vi "DAQmx Task State Model Benchmark.vi"() -> ()   [LabVIEW 2010]
doc: "Description:\nThis VI explores the differences in timing within a VI depending on how the DAQmx Task State is set before running a DAQmx Read VI.\n\nInstructions:\n1. Set the physical channels control to any analog input channel\n2. Run the VI\n3. Observe the different amounts of time the DAQmx Read takes depending upon which State the DAQmx Task was in before the read operation."
uses:
  DAQmx Task States.ctl
  <vilib>/DAQmx/read.llb/DAQmx Read (Analog 1D DBL 1Chan NSamp).vi
  <vilib>/DAQmx/create/channels.llb/DAQmx Create Channel (AI-Voltage-Basic).vi
  <vilib>/daqmx/miscellaneous.llb/DAQmx Fill In Error Info.vi
panel:
  out "Running Task Progress":i32(slide) scale=0.0..100.0
  out "Running Task (ms/iteration)":dbl max=10.0 format="%.2f"
  out "Committed Task Progress":i32(slide) scale=0.0..100.0
  out "Committed Task (ms/iteration)":dbl max=10.0 format="%.2f"
  out "Reserved Task Progress":i32(slide) scale=0.0..100.0
  out "Reserved Task (ms/iteration)":dbl max=10.0 format="%.2f"
  out "Verified Task Progress":i32(slide) scale=0.0..100.0
  out "Verified Task (ms/iteration)":dbl max=10.0 format="%.2f"
  in  "Iterations":i32=100
  out "Unverified Task Progress":i32(slide) scale=0.0..100.0
  out "Unverified Task (ms/iteration)":dbl max=10.0 format="%.2f"
  in  "physical channels":tag
  # "Directions:\n1.  Set the physical channels control to any analog input channel\n2.  Set the number of iterations to the desired number (10 < i < 1000)\n3.  Run the VI\n4.  Observe the difference in execution times depending upon which DAQmx Task State is set before the DAQmx Read.\n\nNote: Each DAQmx Read must continue throught the DAQmx Task States and get to Running before any data can be returned."
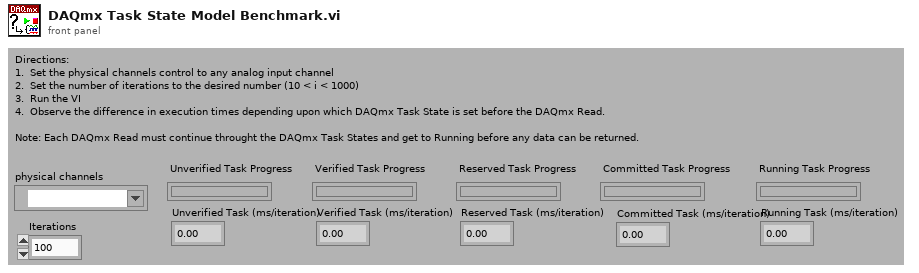
[diagram p1: front panel]
types:
  T1 = typedef "DAQmx Task States.ctl" = enum16{"Unverified", "Verified", "Reserved", "Committed", "Running"}
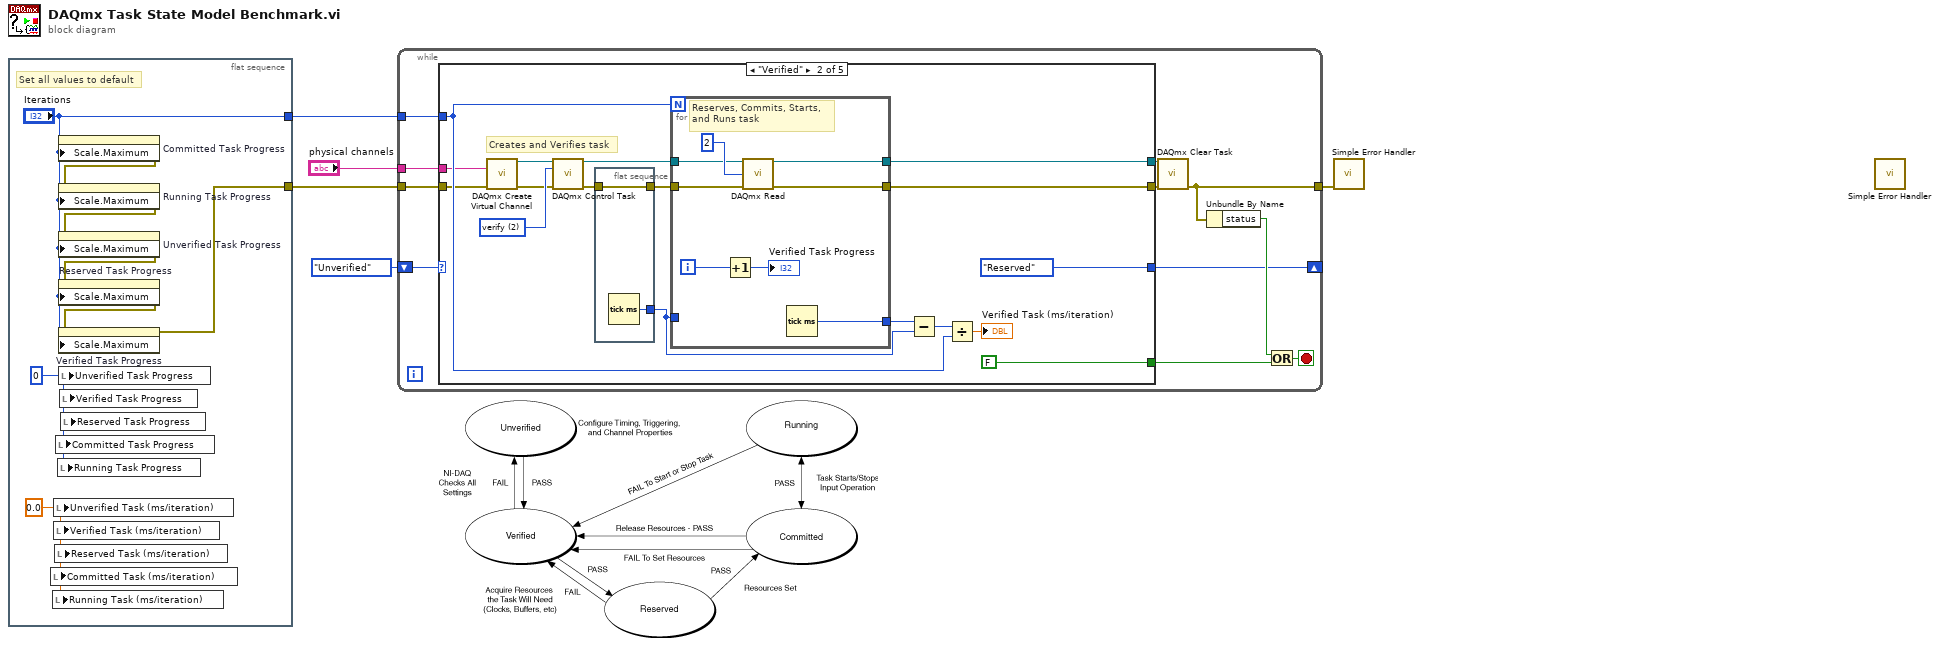
[diagram p0: block diagram]
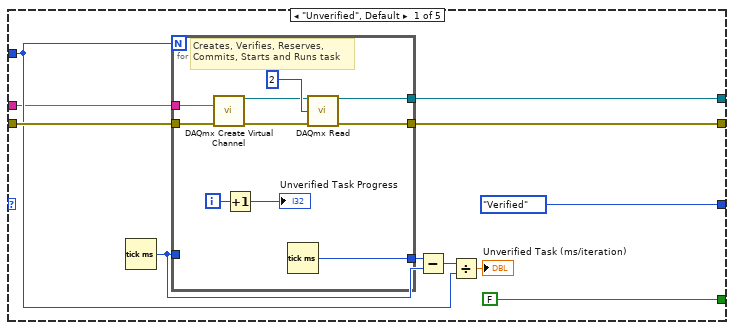
[diagram p2: hidden frame]
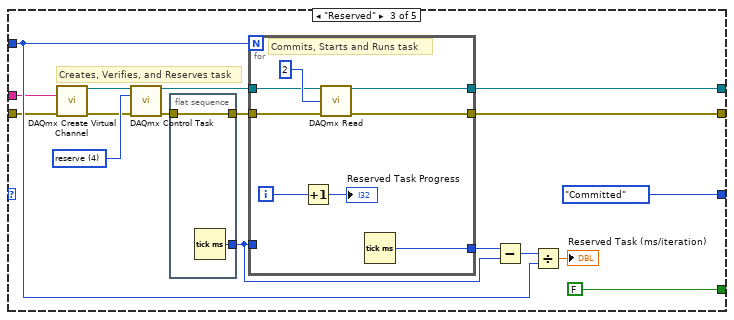
[diagram p3: hidden frame]
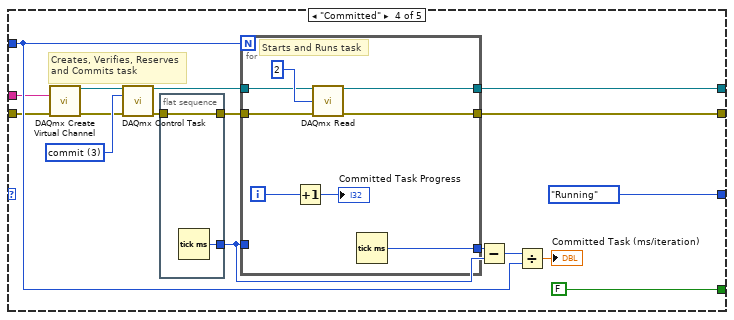
[diagram p4: hidden frame]
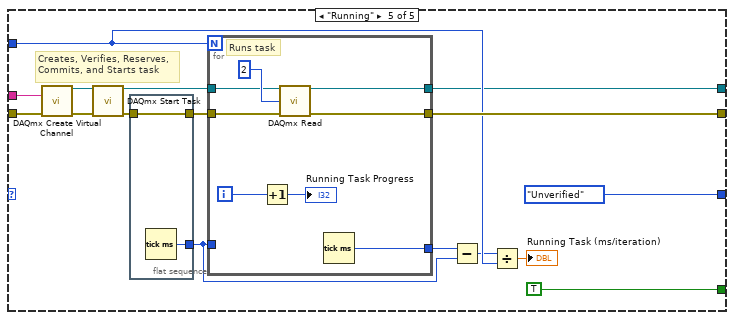
[diagram p5: hidden frame]
diagram:
  n1 = flat-sequence {
    tunnel: ["Iterations"] -> w5
    tunnel: [w7] -> w1
    frame #0 {
      w6 = 0.0 ("Implicit Task (ms/iteration)")
      w13 = 0 ("Implicit")
      # "Set all values to default"
      n2 = local write "Committed Task (ms/iteration)"(w6) -> ()
      n3 = local write "Running Task (ms/iteration)"(w6) -> ()
      n4 = local write "Unverified Task (ms/iteration)"(w6) -> ()
      n5 = local write "Verified Task (ms/iteration)"(w6) -> ()
      n6 = local write "Reserved Task (ms/iteration)"(w6) -> ()
      n7 = local write "Committed Task Progress"(w13) -> ()
      n8 = local write "Running Task Progress"(w13) -> ()
      n9 = property on="Committed Task Progress" class="Gliss (strict)"("Scale.Maximum"="Iterations") -> (error out=w8:errorcluster)  [unwired: 2 in, 1 out]
      n10 = property on="Running Task Progress" class="Gliss (strict)"(error in=w8, "Scale.Maximum"="Iterations") -> (error out=w9:errorcluster)  [unwired: 1 in, 1 out]
      n11 = property on="Unverified Task Progress" class="Gliss (strict)"(error in=w9, "Scale.Maximum"="Iterations") -> (error out=w10:errorcluster)  [unwired: 1 in, 1 out]
      n12 = property on="Reserved Task Progress" class="Gliss (strict)"(error in=w10, "Scale.Maximum"="Iterations") -> (error out=w11:errorcluster)  [unwired: 1 in, 1 out]
      n13 = property on="Verified Task Progress" class="Gliss (strict)"(error in=w11, "Scale.Maximum"="Iterations") -> (error out=w7:errorcluster)  [unwired: 1 in, 1 out]
      n14 = local write "Unverified Task Progress"(w13) -> ()
      n15 = local write "Verified Task Progress"(w13) -> ()
      n16 = local write "Reserved Task Progress"(w13) -> ()
    }
  }
  n17 = while {
    tunnel: w1 -> [w24]
    tunnel: w5 -> [w23]
    shift-right: [w14] -> _
    shift-left: DAQmx_Task_States."Unverified" ("States") -> [w22]
    tunnel: [w15] -> w3
    tunnel: "physical channels" -> [w17]
    stop <- w19 stop-if-true
    n18 = case shown="\"Verified\"" w22 {
      tunnel: w24 -> [w35 w48 w77 w103 w130]
      tunnel: w23 -> [w34 w60 w88 w114 w140]
      tunnel: [FALSE FALSE FALSE FALSE TRUE] -> w18
      tunnel: [w32 w61 w86 w113 w141] -> w16
      tunnel: [w31 w59 w87 w112 w139] -> w21
      tunnel: w17 -> [w26 w47 w74 w101 w128]
      tunnel: [DAQmx_Task_States."Verified" ("States") DAQmx_Task_States."Reserved" ("States") DAQmx_Task_States."Committed" ("States") DAQmx_Task_States."Running" ("States") DAQmx_Task_States."Unverified" ("States")] -> w14
      frame "Unverified", Default {
        n19 = Tick Count (ms)() -> (millisecond timer value=w29:u32)
        n20 = for {
          N: w34 -> [_]
          tunnel: w29 -> [_]
          tunnel: [w45] -> w30
          tunnel: w35 -> [w38]
          tunnel: [w44] -> w32
          tunnel: [w41] -> w31
          tunnel: w26 -> [w36]
          i -> [w43]
          # "Creates, Verifies, Reserves, \nCommits, Starts and Runs task"
          n21 = call-poly <vilib>:"DAQmx Create Virtual Channel.vi"("physical channels"=w36, "error in"=w38) -> ("task out"=w39:refnum<k21>, "error out"=w37:errorcluster)  [unwired: 12 in]
          n22 = Increment(x=w43) -> (x+1=→"Unverified Task Progress":i32)
          n23 = Tick Count (ms)() -> (millisecond timer value=w45:u32)
          n24 = call-poly <vilib>:"DAQmx Read.vi"("task/channels in"=w39, "number of samples per channel"=2, "error in"=w37) -> ("task out"=w41:refnum<k21>, "error out"=w44:errorcluster)  [unwired: 10 in, 1 out]
        }
        n25 = Subtract(x=w30, y=w29) -> (x-y=w28:u32)
        n26 = Divide(x=w28, y=w34) -> (x/y=→"Unverified Task (ms/iteration)":dbl)
      }
      frame "Verified" {
        w57 = 2 items=["verify"=2, "reserve"=4, "commit"=3, "unreserve"=5, "abort"=6] ("action")
        # "Creates and Verifies task"
        n27 = call-poly <vilib>:"DAQmx Create Virtual Channel.vi"("physical channels"=w47, "error in"=w48) -> ("task out"=w50:refnum<k21>, "error out"=w49:errorcluster)  [unwired: 12 in]
        n28 = call <vilib>:"DAQmx Control Task.vi"("task/channels in"=w50, "action"=w57, "error in"=w49) -> ("task out"=w62:refnum<k21>, "error out"=w52:errorcluster)  [unwired: 11 in]
        n29 = flat-sequence {
          tunnel: [w64] -> w56
          tunnel: w52 -> [w63]
          tunnel: [w63] -> w51
          frame #0 {
            n30 = Tick Count (ms)() -> (millisecond timer value=w64:u32)
          }
        }
        n31 = for {
          N: w60 -> [_]
          tunnel: w56 -> [_]
          tunnel: [w71] -> w55
          tunnel: w62 -> [w70]
          tunnel: w51 -> [w69]
          tunnel: [w68] -> w61
          tunnel: [w65] -> w59
          i -> [w67]
          # "Reserves, Commits, Starts, \nand Runs task"
          n32 = Increment(x=w67) -> (x+1=→"Verified Task Progress":i32)
          n33 = call-poly <vilib>:"DAQmx Read.vi"("task/channels in"=w70, "number of samples per channel"=2, "error in"=w69) -> ("task out"=w65:refnum<k21>, "error out"=w68:errorcluster)  [unwired: 10 in, 1 out]
          n34 = Tick Count (ms)() -> (millisecond timer value=w71:u32)
        }
        n35 = Subtract(x=w55, y=w56) -> (x-y=w54:u32)
        n36 = Divide(x=w54, y=w60) -> (x/y=→"Verified Task (ms/iteration)":dbl)
      }
      frame "Reserved" {
        w84 = 4 items=["verify"=2, "reserve"=4, "commit"=3, "unreserve"=5, "abort"=6] ("action")
        # "Creates, Verifies, and Reserves task"
        n37 = call-poly <vilib>:"DAQmx Create Virtual Channel.vi"("physical channels"=w74, "error in"=w77) -> ("task out"=w75:refnum<k21>, "error out"=w76:errorcluster)  [unwired: 12 in]
        n38 = call <vilib>:"DAQmx Control Task.vi"("task/channels in"=w75, "action"=w84, "error in"=w76) -> ("task out"=w89:refnum<k21>, "error out"=w78:errorcluster)  [unwired: 11 in]
        n39 = flat-sequence {
          tunnel: [w91] -> w83
          tunnel: [w90] -> w79
          tunnel: w78 -> [w90]
          frame #0 {
            n40 = Tick Count (ms)() -> (millisecond timer value=w91:u32)
          }
        }
        n41 = for {
          N: w88 -> [_]
          tunnel: w83 -> [_]
          tunnel: [w98] -> w82
          tunnel: w89 -> [w97]
          tunnel: w79 -> [w96]
          tunnel: [w95] -> w86
          tunnel: [w92] -> w87
          i -> [w94]
          # "Commits, Starts and Runs task"
          n42 = Increment(x=w94) -> (x+1=→"Reserved Task Progress":i32)
          n43 = call-poly <vilib>:"DAQmx Read.vi"("task/channels in"=w97, "number of samples per channel"=2, "error in"=w96) -> ("task out"=w92:refnum<k21>, "error out"=w95:errorcluster)  [unwired: 10 in, 1 out]
          n44 = Tick Count (ms)() -> (millisecond timer value=w98:u32)
        }
        n45 = Subtract(x=w82, y=w83) -> (x-y=w81:u32)
        n46 = Divide(x=w81, y=w88) -> (x/y=→"Reserved Task (ms/iteration)":dbl)
      }
      frame "Committed" {
        w111 = 3 items=["verify"=2, "reserve"=4, "commit"=3, "unreserve"=5, "abort"=6] ("action")
        # "Creates, Verifies, Reserves\nand Commits task"
        n47 = call-poly <vilib>:"DAQmx Create Virtual Channel.vi"("physical channels"=w101, "error in"=w103) -> ("task out"=w102:refnum<k21>, "error out"=w104:errorcluster)  [unwired: 12 in]
        n48 = call <vilib>:"DAQmx Control Task.vi"("task/channels in"=w102, "action"=w111, "error in"=w104) -> ("task out"=w115:refnum<k21>, "error out"=w105:errorcluster)  [unwired: 11 in]
        n49 = flat-sequence {
          tunnel: [w118] -> w110
          tunnel: [w117] -> w106
          tunnel: w105 -> [w117]
          frame #0 {
            n50 = Tick Count (ms)() -> (millisecond timer value=w118:u32)
          }
        }
        n51 = for {
          N: w114 -> [_]
          tunnel: w110 -> [_]
          tunnel: [w125] -> w109
          tunnel: w115 -> [w124]
          tunnel: w106 -> [w123]
          tunnel: [w122] -> w113
          tunnel: [w119] -> w112
          i -> [w121]
          # "Starts and Runs task"
          n52 = Increment(x=w121) -> (x+1=→"Committed Task Progress":i32)
          n53 = call-poly <vilib>:"DAQmx Read.vi"("task/channels in"=w124, "number of samples per channel"=2, "error in"=w123) -> ("task out"=w119:refnum<k21>, "error out"=w122:errorcluster)  [unwired: 10 in, 1 out]
          n54 = Tick Count (ms)() -> (millisecond timer value=w125:u32)
        }
        n55 = Subtract(x=w109, y=w110) -> (x-y=w108:u32)
        n56 = Divide(x=w108, y=w114) -> (x/y=→"Committed Task (ms/iteration)":dbl)
      }
      frame "Running" {
        # "Creates, Verifies, Reserves, \nCommits, and Starts task"
        n57 = call-poly <vilib>:"DAQmx Create Virtual Channel.vi"("physical channels"=w128, "error in"=w130) -> ("task out"=w131:refnum<k21>, "error out"=w129:errorcluster)  [unwired: 12 in]
        n58 = call <vilib>:"DAQmx Start Task.vi"("task/channels in"=w131, "error in"=w129) -> ("task out"=w142:refnum<k21>, "error out"=w133:errorcluster)  [unwired: 12 in]
        n59 = flat-sequence {
          tunnel: [w144] -> w137
          tunnel: w133 -> [w143]
          tunnel: [w143] -> w132
          frame #0 {
            n60 = Tick Count (ms)() -> (millisecond timer value=w144:u32)
          }
        }
        n61 = for {
          N: w140 -> [_]
          tunnel: w137 -> [_]
          tunnel: [w151] -> w136
          tunnel: w142 -> [w150]
          tunnel: w132 -> [w149]
          tunnel: [w148] -> w141
          tunnel: [w145] -> w139
          i -> [w147]
          # "Runs task"
          n62 = Increment(x=w147) -> (x+1=→"Running Task Progress":i32)
          n63 = call-poly <vilib>:"DAQmx Read.vi"("task/channels in"=w150, "number of samples per channel"=2, "error in"=w149) -> ("task out"=w145:refnum<k21>, "error out"=w148:errorcluster)  [unwired: 10 in, 1 out]
          n64 = Tick Count (ms)() -> (millisecond timer value=w151:u32)
        }
        n65 = Subtract(x=w136, y=w137) -> (x-y=w135:u32)
        n66 = Divide(x=w135, y=w140) -> (x/y=→"Running Task (ms/iteration)":dbl)
      }
    }
    n67 = call <vilib>:"DAQmx Clear Task.vi"("task in"=w21, "error in"=w16) -> ("error out"=w15:errorcluster)  [unwired: 13 in]
    n68 = Unbundle By Name(w15) -> ("status"=w20:bool)
    n69 = Or(x=w20, y=w18) -> (x .or. y?=w19:bool)
  }
  n70 = call <vilib>:"Simple Error Handler.vi"("error in (no error)"=w3) -> ()  [unwired: 4 in, 5 out]
  n71 = call <vilib>:"Simple Error Handler.vi"() -> ()  [unwired: 5 in, 5 out]
